vi "Hz to Ms.vi"(11 "Value":dbl) -> (3 "Timing Parameters":T1)   [LabVIEW 2024, in "Sift Stream.lvlib" / "Sift Stream.lvclass"]
uses:
  Sift Stream.lvclass
  <vilib>/FlexLogger/SDK/PluginSDK.lvlibp/PEFClasses/SDK/Processing Element/Timing Parameters.ctl
  <vilib>/FlexLogger/SDK/PluginSDK.lvlibp/PEFClasses/SDK/Processing Element/Timing Method.ctl
  <vilib>/FlexLogger/SDK/PluginSDK.lvlibp/PEFClasses/SDK/Processing Element/Processing Element.lvclass
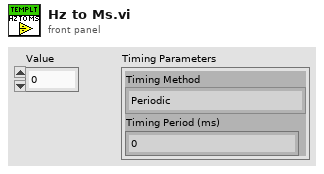
[diagram p1: front panel]
types:
  T1 = typedef "PluginSDK.lvlibp/Processing Element.lvclass/Timing Parameters.ctl" = cluster{"Timing Method":T2, "Timing Period (ms)":i32}
  T2 = typedef "PluginSDK.lvlibp/Processing Element.lvclass/Timing Method.ctl" = enum16{"Periodic", "Immediate", "On Data Ready", "Triggered"}
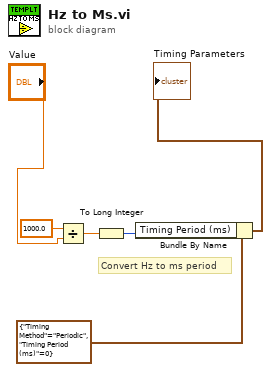
[diagram p0: block diagram]
diagram:
  # "Convert Hz to ms period"
  n1 = Divide(x=1000.0, y="Value") -> (x/y=w2:dbl)
  n2 = To Long Integer(number=w2) -> (32bit integer=w5:i32)
  n3 = Bundle By Name(cluster=T1 {"Timing Method"=enum."Periodic", "Timing Period (ms)"=0} ("Timing Parameters"), "Timing Period (ms)"=w5) -> (→"Timing Parameters":T1)
